vi "prepare image for 2nd mom analysis.vi"(8 "error in (no error)":errorcluster, 11 "FakeCamera in":refnum<class "Point Grey Camera.lvclass">) -> (0 "error out":errorcluster, 2 "BG sub image":T1(plugin-control), 3 "thresholded for 2nd mom":T1, 5 "FakeCamera out":refnum<class "Point Grey Camera.lvclass">)   [LabVIEW 2020, in "Point Grey Camera.lvclass"]
uses:
  Point Grey Camera.lvclass
  IMAQ Image.ctl
  Point Grey Camera.lvclass/Point Grey Camera.ctl
  NI_Vision_Development_Module.lvlib
panel:
  out "thresh for 2nd mom out":T1
  out "BG sub image 45":T1(plugin-control)
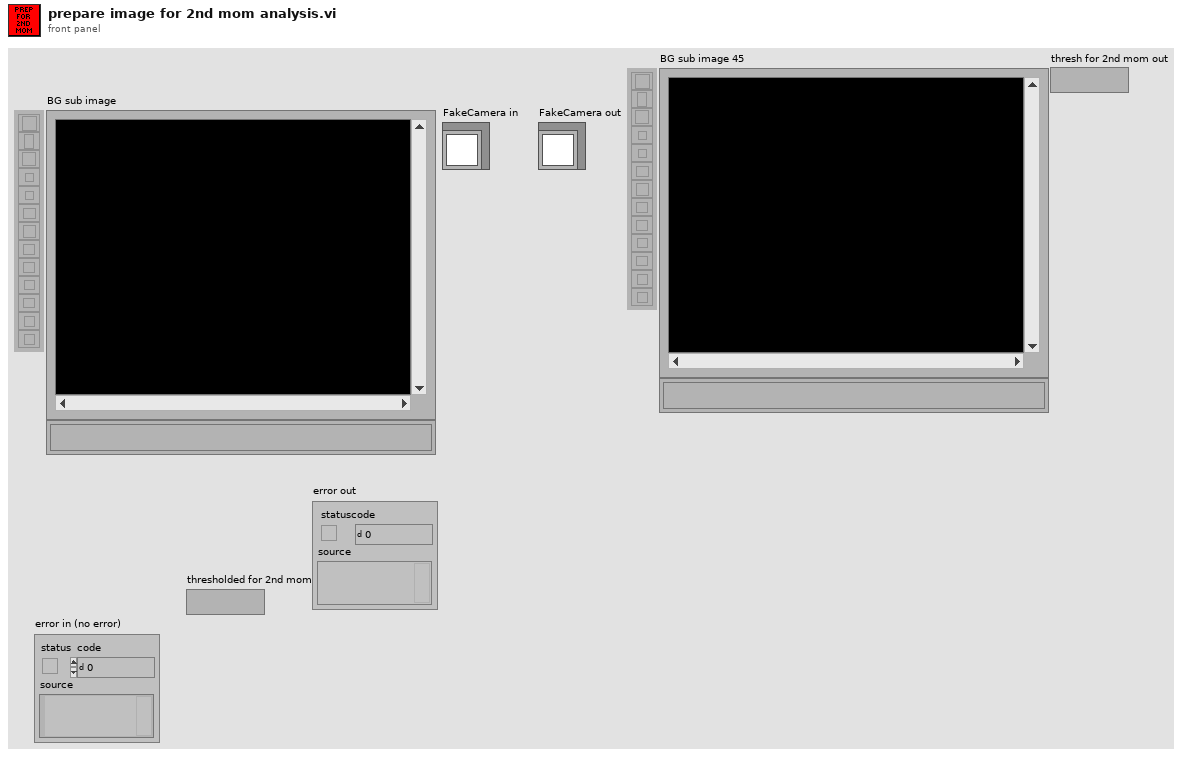
[diagram p1: front panel]
types:
  T1 = typedef "IMAQ Image.ctl" = refnum<image>
  T2 = typedef "Image Type" = u32
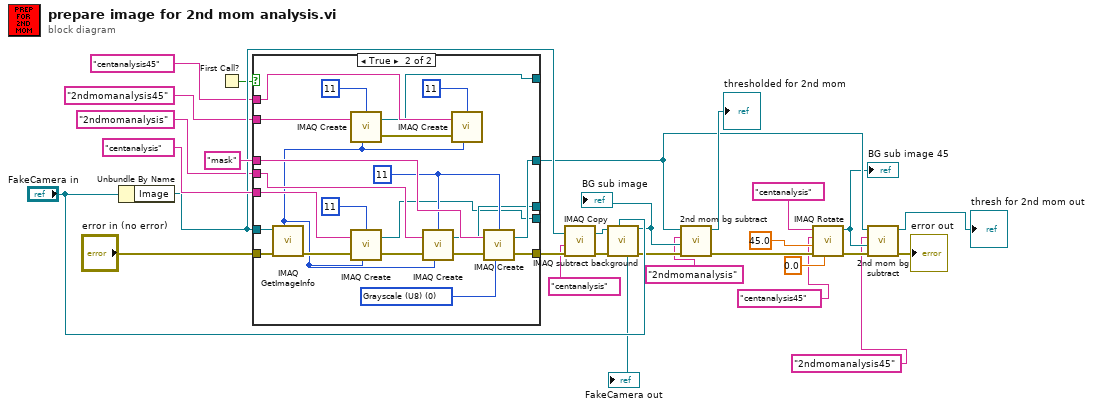
[diagram p0: block diagram]
diagram:
  n1 = Unbundle By Name("FakeCamera in") -> ("Image"=w25:T1)
  n2 = First Call?() -> (First Call?: T/F=w21:bool)
  n3 = case shown="True" w21 {
    tunnel: [w34 w56] -> w12
    tunnel: "mask" ("Image Name") -> [w34 w54]
    tunnel: "centanalysis" ("Image Name") -> [w32 w50]
    tunnel: "error in (no error)" -> [w31 w46]
    tunnel: w25 -> [_ w48]
    tunnel: "2ndmomanalysis" ("Image Name") -> [w33 w47]
    tunnel: [w31 w45] -> w18
    tunnel: [w33 w44] -> _
    tunnel: [w32 w43] -> _
    tunnel: "2ndmomanalysis45" ("Image Name") -> [w30 w40]
    tunnel: "centanalysis45" ("Image Name") -> [_ w38]
    tunnel: [w30 w36] -> _
    frame False {
    }
    frame True {
      w55 = T2 0 items=["Grayscale (U8)", "Grayscale (I16)", "Grayscale (SGL)", "Complex (CSG)", "RGB (U32)", "HSL (U32)", "RGB (U64)", "Grayscale (U16)"] ("Image Type")
      w49 = 11 ("Border Size")
      n4 = call "IMAQ GetImageInfo"("error in (no error)"=w46, "Image"=w48) -> ("error out"=w52:errorcluster, "Image Type"=w35:T2)  [unwired: 2 in, 6 out]
      n5 = call "IMAQ Create"("Border Size"=11, "Image Name"=w40, "Image Type"=w35) -> ("New Image"=w36:T1, "error out"=w37:errorcluster)  [unwired: 2 in]
      n6 = call "IMAQ Create"("Border Size"=11, "Image Name"=w50, "Image Type"=w35, "error in (no error)"=w52) -> ("New Image"=w43:T1, "error out"=w42:errorcluster)  [unwired: 1 in]
      n7 = call "IMAQ Create"("Border Size"=w49, "Image Name"=w47, "Image Type"=w35, "error in (no error)"=w42) -> ("New Image"=w44:T1, "error out"=w53:errorcluster)  [unwired: 1 in]
      n8 = call "IMAQ Create"("Border Size"=11, "Image Name"=w38, "Image Type"=w35, "error in (no error)"=w37) -> ()  [unwired: 1 in, 2 out]
      n9 = call "IMAQ Create"("Border Size"=w49, "Image Name"=w54, "Image Type"=w55, "error in (no error)"=w53) -> ("New Image"=w56:T1, "error out"=w45:errorcluster)  [unwired: 1 in]
    }
  }
  n10 = call "IMAQ Copy"("error in (no error)"=w18, "Image Dst"="centanalysis" ("Image Name"), "Image Src"=w25) -> ("error out"=w20:errorcluster, "Image Dst Out"=w19:T1)  [unwired: 3 in]
  n11 = call "IMAQ subtract background.vi"("FakeCamera in"="FakeCamera in", "error in (no error)"=w20, "Image in"=w19) -> ("error out"=w9:errorcluster, "Refnum out"=w13:T1, "FakeCamera out"=→"FakeCamera out":refnum<class "Point Grey Camera.lvclass">)  [unwired: 3 in, 3 out]
  "BG sub image" <- w13
  n12 = call "2nd mom bg subtract.vi"("error in (no error)"=w9, "BG sub in"=w13, "2ndmom"="2ndmomanalysis" ("Image Name"), "mask"=w12) -> ("error out"=w8:errorcluster, "thresh for 2nd mom out"=→"thresholded for 2nd mom":T1)  [unwired: 6 in]
  n13 = call "IMAQ Rotate"("Replace Value"=sgl 0.0, "error in (no error)"=w8, "Angle (degrees)"=sgl 45.0, "Image Dst"="centanalysis45" ("Image Name"), "Image Src"="centanalysis" ("Image Name")) -> ("error out"=w7:errorcluster, "Image Dst Out"=w11:T1)  [unwired: 5 in]
  "BG sub image 45" <- w11
  n14 = call "2nd mom bg subtract.vi"("error in (no error)"=w7, "BG sub in"=w11, "2ndmom"="2ndmomanalysis45" ("Image Name"), "mask"=w12) -> ("error out"=→"error out":errorcluster, "thresh for 2nd mom out"=→"thresh for 2nd mom out":T1)  [unwired: 6 in]
